vi "setInputFilenameReplacement.vi"(8 "error in (no error)":errorcluster, 10 "replacementPattern":string, 11 "VGS_Job in":refnum<class "VGS_Job.lvclass">) -> (0 "error out":errorcluster, 3 "VGS_Job out":refnum<class "VGS_Job.lvclass">)   [LabVIEW 2022 SP3, in "LV_VGS.lvlib" / "VGS_Job.lvclass"]
uses:
  VGS_Job.lvclass
  VGS_Job.lvclass/VGS_Job.ctl
  C:/Users/Andrey/Documents/GitHub/LV_VGS/vgs_project.dll
  vgs_project.dll
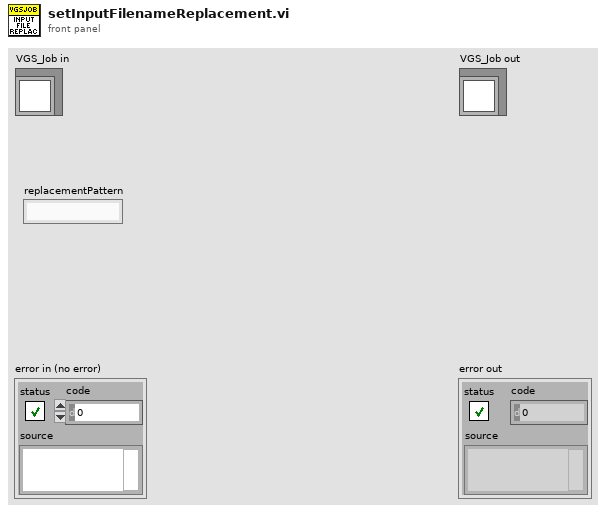
[diagram p1: front panel]
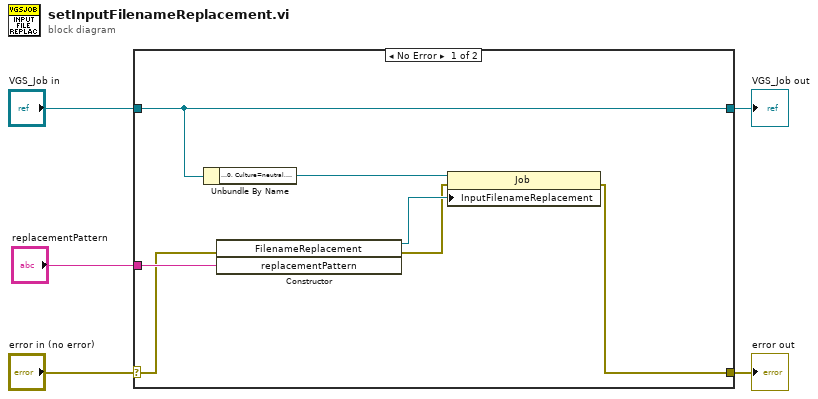
[diagram p0: block diagram]
diagram:
  n1 = case shown="No Error" "error in (no error)" {
    selector: "error in (no error)" -> [w8 w14]
    tunnel: [w6 w14] -> w4
    tunnel: [w12 w13] -> w2
    tunnel: "VGS_Job in" -> [w12 w13]
    tunnel: "replacementPattern" -> [w9 _]
    frame No Error {
      n2 = Unbundle By Name(w12) -> ("Job reference"=w11:refnum<k24>)
      n3 = constructor class="Job+FilenameReplacement"(error in=w8, "replacementPattern"=w9) -> (reference out=w10:refnum<k24>, error out=w7:errorcluster)  [unwired: 2 in, 2 out]
      n4 = property class="Job"(reference=w11, error in=w7, "InputFilenameReplacement"=w10) -> (error out=w6:errorcluster)  [unwired: 1 out]
    }
    frame Error {
    }
  }
  "error out" <- w4
  "VGS_Job out" <- w2
